vi "Config AFE.vi"(10 "dc (T) altern (F)":bool) -> (2 "OK":bool)   [LabVIEW 2019]
uses:
  <vilib>/Utility/file.llb/Read Delimited Spreadsheet (string).vi
  <vilib>/Modbus/master/Create Master Instance (Serial).vi
  <vilib>/Modbus/master/Modbus Master.lvclass
panel:
  out "register values 2":u16[](array[numeric])
  out "register values":u16[](array[numeric])
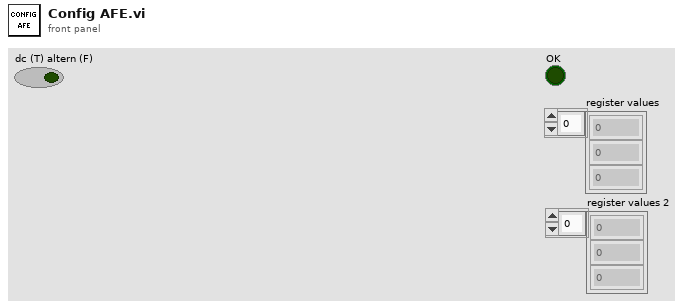
[diagram p1: front panel]
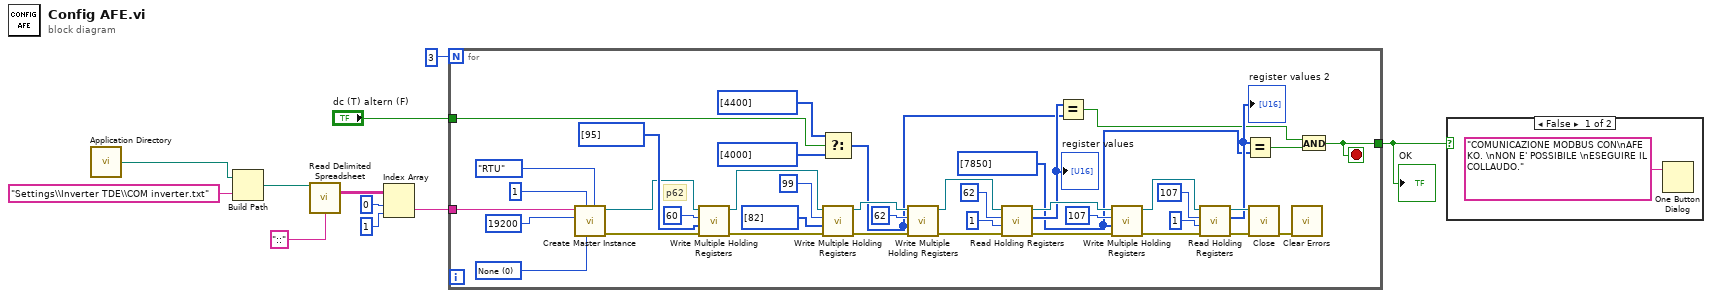
[diagram p0: block diagram]
diagram:
  n1 = call <vilib>:"Application Directory.vi"() -> ("Application Directory"=w8:path)
  n2 = Build Path(base path=w8, name or relative path="Settings\\Inverter TDE\\COM inverter.txt") -> (appended path=w7:path)
  n3 = call-poly <vilib>:"Read Delimited Spreadsheet.vi"("file path (dialog if empty)"=w7, "delimiter (\\t)"="::" ("delimiter (\\t)")) -> ("all rows"=w4:string[][])  [unwired: 8 in, 5 out]
  n4 = Index Array(array=w4, index (row)=0 ("disabled index (row)"), index (col)=1 ("disabled index (col)")) -> (element=w1:string)
  n5 = for {
    N: 3 -> [_]
    tunnel: [w15] -> w10
    tunnel: "dc (T) altern (F)" -> [w14]
    tunnel: w1 -> [w12]
    stop <- w15 stop-if-true
    w18 = u16[] [7850] ("holding register values")
    w46 = u16 0 items=["None", "Odd", "Even"] ("parity (Even)")
    # "p62"
    n6 = call-poly <vilib>:"Create Master Instance.vi"("serial type"=enum16{"RTU", "ASCII"}."RTU", "parity (Even)"=w46, "unit ID"=u8 1, "baud rate (9600)"=u32 19200, "VISA resource name"=w12) -> ("error out"=w43:errorcluster, "serial master instance"=w44:refnum<class "Modbus Master.lvclass">)  [unwired: 5 in]
    n7 = call-dynamic "Write Multiple Holding Registers.vi"("error in (no error)"=w43, "holding register values"=u16[] [95], "starting address"=u16 60, "Modbus master in"=w44) -> ("error out"=w26:errorcluster, "Modbus master out"=w28:refnum<class "Modbus Master.lvclass">)  [unwired: 6 in]
    n8 = Select(t=u16[] [4400] ("holding register values"), s=w14, f=u16[] [4000] ("holding register values")) -> (s? t:f=w20:u16[])
    n9 = call-dynamic "Write Multiple Holding Registers.vi"("error in (no error)"=w26, "holding register values"=u16[] [82], "starting address"=u16 99, "Modbus master in"=w28) -> ("error out"=w25:errorcluster, "Modbus master out"=w27:refnum<class "Modbus Master.lvclass">)  [unwired: 6 in]
    n10 = call-dynamic "Write Multiple Holding Registers.vi"("error in (no error)"=w25, "holding register values"=w20, "starting address"=u16 62, "Modbus master in"=w27) -> ("error out"=w41:errorcluster, "Modbus master out"=w39:refnum<class "Modbus Master.lvclass">)  [unwired: 6 in]
    n11 = call-dynamic "Read Holding Registers.vi"("error in (no error)"=w41, "number of holding registers"=u16 1, "starting address"=u16 62, "Modbus master in"=w39) -> ("error out"=w33:errorcluster, "register values"=w21:u16[], "Modbus master out"=w35:refnum<class "Modbus Master.lvclass">)  [unwired: 5 in]
    "register values" <- w21
    n12 = Equal?(x=w21, y=w20) -> (x = y?=w16:bool)
    n13 = call-dynamic "Write Multiple Holding Registers.vi"("error in (no error)"=w33, "holding register values"=w18, "starting address"=u16 107, "Modbus master in"=w35) -> ("error out"=w32:errorcluster, "Modbus master out"=w34:refnum<class "Modbus Master.lvclass">)  [unwired: 6 in]
    n14 = call-dynamic "Read Holding Registers.vi"("error in (no error)"=w32, "number of holding registers"=u16 1, "starting address"=u16 107, "Modbus master in"=w34) -> ("error out"=w31:errorcluster, "register values"=w19:u16[], "Modbus master out"=w37:refnum<class "Modbus Master.lvclass">)  [unwired: 5 in]
    "register values 2" <- w19
    n15 = Equal?(x=w19, y=w18) -> (x = y?=w17:bool)
    n16 = call-dynamic "Close.vi"("error in (no error)"=w31, "Modbus master in"=w37) -> ("error out"=w13:errorcluster)  [unwired: 9 in]
    n17 = call <vilib>:"Clear Errors.vi"("error in (no error)"=w13) -> ()  [unwired: 5 in, 2 out]
    n18 = And(x=w16, y=w17) -> (x .and. y?=w15:bool)
  }
  "OK" <- w10
  n19 = case shown="False" w10 {
    frame False {
      n20 = One Button Dialog(message="COMUNICAZIONE MODBUS CON\nAFE KO. \nNON E' POSSIBILE \nESEGUIRE IL COLLAUDO.") -> ()  [unwired: 1 in, 1 out]
    }
    frame True {
    }
  }
